vi "Keithley DMM6500 DAQ6500 Series Scanning Temperature With Thermocouples.vi"() -> ()   [LabVIEW 2023]
doc: "This example shows how to scan temperature with thermocouples"
uses:
  <instrlib>/Keithley DMM6500 DAQ6500 Series/Public/Configure/Configure Temperature (Thermocouple).vi
  <instrlib>/Keithley DMM6500 DAQ6500 Series/Public/Data/Read (Multiple Points).vi
  <instrlib>/Keithley DMM6500 DAQ6500 Series/Keithley DMM6500 DAQ6500 Series.lvlib
panel:
  in  "Buffer Element2 ()":i32(ring) items=["", "Date", "Extra", "Formatted", "Fractional", "Reading", "Relative", "Seconds", "Status", "Time", "Tstamp", "Unit", "CHAN", "Extra Form", "Extra Unit"]
  in  "Buffer Element1 ()":i32(ring) items=["", "Date", "Extra", "Formatted", "Fractional", "Reading", "Relative", "Seconds", "Status", "Time", "Tstamp", "Unit", "CHAN", "Extra Format", "Extra Unit"]
  in  "File Name(\"/usb1/scan24hr.csv\")":string="/usb1/scan24hr.csv"
  out "Measurements":dbl[](array[numeric])
  in  "Reference Junction Type (1: Internal)":i32(ring)=1 items=["Simulated", "Internal", "External"]
  in  "Thermocouple Type (3: K)":i32(ring)=3 items=["B", "E", "J", "K", "N", "R", "S", "T"]
  in  "Unit (1: Celsius)":i32(ring)=1 items=["Kelvin", "Celsius", "Fahrenheit"]
  in  "Reading Buffer Size (14400)":u32=14400
  in  "Reading Buffer (\"defbuffer1\")":string="defbuffer1"
  in  "Scan Interval (60 s)":dbl=60.0
  in  "Scan Count (1440)":u32=1440
  in  "Channel List (\"101:110\")":string="101:110"
  in  "VISA resource name":refnum<visa-resource-name>
  # "(c) 2018-2022 National Instruments.  ALL RIGHTS RESERVED."
  # "This example VI demonstrates how to use the DAQ6500 Series to log thermocouple-based temperature\nmeasurement scans using internal cold-junction compensation (CJC) correction over a 24-hour period."
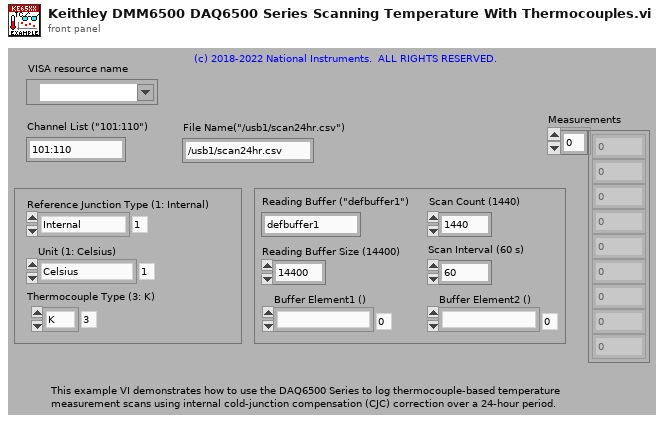
[diagram p1: front panel]
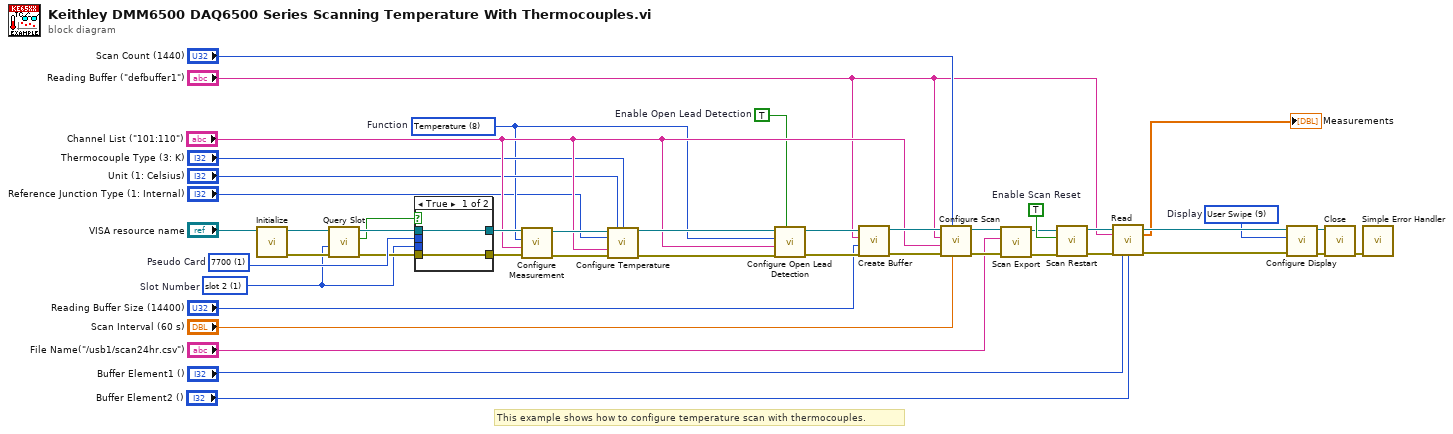
[diagram p0: block diagram]
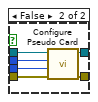
[diagram p2: hidden frame]
diagram:
  w16 = 9 items=["Home Screen", "Home with Large Readings", "Reading Table", "Graph", "Functions Swipe", "Graph Swipe", "Secondary Swipe", "Setting Swipe", "Statistic Swipe", "User Swipe", "Channel Swipe", "Nonswich Swipe", "Scan Swipe", "Control Channel", "Settings Channel", "Scan Channel"]  # Display
  w12 = 1 items=["slot 1", "slot 2"]  # Slot Number
  w32 = 1 items=["0", "7700", "7701", "7702", "7703", "7705", "7706", "7707", "7708", "7709", "7710", "7711", "7712"]  # Pseudo Card
  w19 = 8 items=[" Voltage DC", "Voltage AC", "Current DC", "Current AC", "Resistance", "4-wire Resistance", "Diode", "Capacitance", "Temperature", "Continuity", "Frequency", "Period", "Voltage Ratio", "Digitize Voltage", "Digitize Current"]  # Function
  w40 = TRUE  # Enable Scan Reset
  w20 = TRUE  # Enable Open Lead Detection
  # "This example shows how to configure temperature scan with thermocouples."
  n1 = call <instrlib>:"Initialize.vi"("VISA resource name"="VISA resource name") -> ("error out"=w14:errorcluster, "VISA resource name out"=w43:refnum<visa-resource-name>)  [unwired: 9 in]
  n2 = call <instrlib>:"Query Slot.vi"("error in (no error)"=w14, "Slot Number(0: slot 1)"=w12, "VISA resource name"=w43) -> ("error out"=w13:errorcluster, "Real Card In Slot"=w11:bool, "VISA resource name out"=w15:refnum<visa-resource-name>)  [unwired: 6 in]
  n3 = case shown="True" w11 {
    tunnel: [w47 w53] -> w42
    tunnel: [w46 w52] -> w41
    tunnel: w32 -> [_ w51]
    tunnel: w15 -> [w47 w50]
    tunnel: w13 -> [w46 w49]
    tunnel: w12 -> [_ w48]
    frame True {
    }
    frame False {
      n4 = call <instrlib>:"Configure Pseudo Card.vi"("error in (no error)"=w49, "Slot Number (0: slot1)"=w48, "Pseudo Card (0:No pseudocard)"=w51, "VISA resource name"=w50) -> ("error out"=w52:errorcluster, "VISA resource name out"=w53:refnum<visa-resource-name>)  [unwired: 6 in]
    }
  }
  n5 = call <instrlib>:"Configure Measurement.vi"("error in (no error)"=w41, "Channel List(\"\")"="Channel List (\"101:110\")", "Function (0: Voltage DC)"=w19, "VISA resource name"=w42) -> ("error out"=w29:errorcluster, "VISA resource name out"=w31:refnum<visa-resource-name>)  [unwired: 6 in]
  n6 = call-poly <instrlib>:"Configure Temperature.vi"("VISA resource name"=w31, "Unit (1: Celsius)"="Unit (1: Celsius)", "Thermocouple Type (3: K)"="Thermocouple Type (3: K)", "Reference Junction Type (1: Internal)"="Reference Junction Type (1: Internal)", "Channel List(\"\")"="Channel List (\"101:110\")", "error in (no error)"=w29) -> ("VISA resource name out"=w30:refnum<visa-resource-name>, "error out"=w28:errorcluster)  [unwired: 8 in]
  n7 = call <instrlib>:"Configure Open Lead Detection.vi"("Enable Open Lead Detection (F: Disable)"=w20, "error in (no error)"=w28, "Channel List(\"\")"="Channel List (\"101:110\")", "Function (5: 4-wire resistance)"=w19, "VISA resource name"=w30) -> ("error out"=w34:errorcluster, "VISA resource name out"=w35:refnum<visa-resource-name>)  [unwired: 5 in]
  n8 = call <instrlib>:"Create Buffer.vi"("error in (no error)"=w34, "Buffer Size (10)"="Reading Buffer Size (14400)", "Buffer Name (\"\")"="Reading Buffer (\"defbuffer1\")", "VISA resource name"=w35) -> ("error out"=w36:errorcluster, "VISA resource name out"=w37:refnum<visa-resource-name>)  [unwired: 6 in]
  n9 = call <instrlib>:"Configure Scan.vi"("Delay Seconds (0 s)"="Scan Interval (60 s)", "Scan Count (1)"="Scan Count (1440)", "error in (no error)"=w36, "Channel List(\"\")"="Channel List (\"101:110\")", "Reading Buffer (\"\")"="Reading Buffer (\"defbuffer1\")", "VISA resource name"=w37) -> ("error out"=w6:errorcluster, "VISA resource name out"=w7:refnum<visa-resource-name>)  [unwired: 4 in]
  n10 = call <instrlib>:"Scan Export.vi"("error in (no error)"=w6, "File Name (\"\")"="File Name(\"/usb1/scan24hr.csv\")", "VISA resource name"=w7) -> ("error out"=w5:errorcluster, "VISA resource name out"=w4:refnum<visa-resource-name>)  [unwired: 7 in]
  n11 = call <instrlib>:"Scan Restart.vi"("error in (no error)"=w5, "Enable Scan Reset (T: Enable)"=w40, "VISA resource name"=w4) -> ("error out"=w23:errorcluster, "VISA resource name out"=w24:refnum<visa-resource-name>)  [unwired: 7 in]
  n12 = call-poly <instrlib>:"Read.vi"("VISA resource name"=w24, "Buffer Name (\"\")"="Reading Buffer (\"defbuffer1\")", "error in (no error)"=w23, "Buffer Element1 ()"="Buffer Element1 ()", "Buffer Element2 ()"="Buffer Element2 ()") -> ("VISA resource name out"=w22:refnum<visa-resource-name>, "Measurements"=→"Measurements":dbl[], "error out"=w9:errorcluster)  [unwired: 8 in]
  n13 = call <instrlib>:"Configure Display.vi"("error in (no error)"=w9, "Display (0: Home Screen)"=w16, "VISA resource name"=w22) -> ("error out"=w8:errorcluster, "VISA resource name out"=w17:refnum<visa-resource-name>)  [unwired: 7 in]
  n14 = call <instrlib>:"Close.vi"("error in (no error)"=w8, "VISA resource name"=w17) -> ("error out"=w45:errorcluster)  [unwired: 9 in]
  n15 = call <vilib>:"Simple Error Handler.vi"("error in (no error)"=w45) -> ()  [unwired: 4 in, 5 out]
